vi "Open Log File.vi"(8 "error in (no error)":errorcluster, 10 "Path":path, 11 "CSV Word Logger in":refnum<class "CSV Word Logger.lvclass">) -> (0 "error out":errorcluster, 3 "CSV Word Logger out":refnum<class "CSV Word Logger.lvclass">)   [LabVIEW 2020, in "Ballard ARINC 429 Engine.lvlib" / "Implementation.lvlib" / "Word Logging.lvlib" / "CSV Word Logger.lvclass"]
uses:
  CSV Word Logger.lvclass
  CSV Word Logger.lvclass/CSV Word Logger.ctl
  351de733-b961-4ed4-9e08-ca322b6c372e.vi
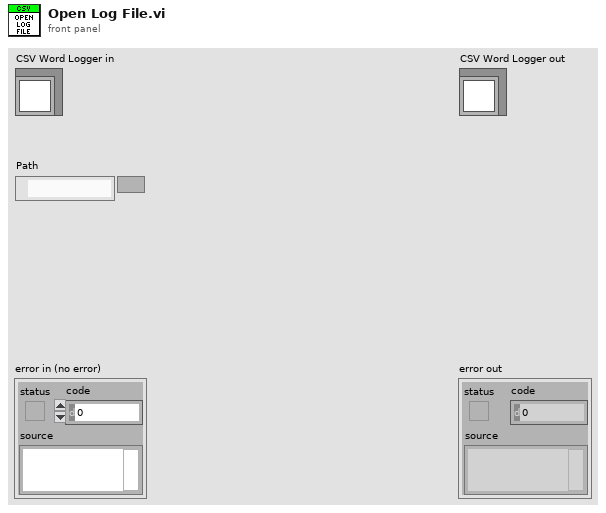
[diagram p1: front panel]
types:
  T1 = enum16{"open", "replace", "create", "open or create", "replace or create", "replace or create with confirmation"}
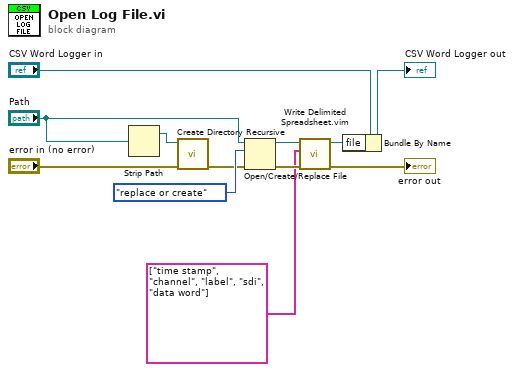
[diagram p0: block diagram]
diagram:
  n1 = Strip Path(path="Path") -> (stripped path=w2:path)  [unwired: 1 out]
  n2 = call <vilib>:"Create Directory Recursive.vi"("error in (no error)"="error in (no error)", "directory"=w2) -> ("error out"=w4:errorcluster)  [unwired: 3 in, 2 out]
  n3 = Open/Create/Replace File(file path (use dialog)="Path", error in=w4, operation (0:open)=T1."replace or create") -> (refnum out=w7:refnum<file>, error out=w9:errorcluster)  [unwired: 3 in, 1 out]
  n4 = call "Write Delimited Spreadsheet.vim"("error in (no error)"=w9, "data"=string[] ["time stamp", "channel", "label", "sdi", "data word"], "file in"=w7) -> ("error out"=→"error out":errorcluster, "file out"=w10:refnum<file>)  [unwired: 7 in]
  n5 = Bundle By Name(cluster="CSV Word Logger in", "file"=w10) -> (→"CSV Word Logger out":refnum<class "CSV Word Logger.lvclass">)
